vi "data to registers.vi"(6 "word order":T1, 9 "specifications":T2[](array[typedef]), 10 "allocation":u16[](array[numeric]), 11 "data table":T4) -> (2 "registers":u16[](array[numeric]), 3 "allocation":T4)   [LabVIEW 2015, in "Modbus Module runtime.lvclass"]
uses:
  Modbus Module runtime.lvclass
  <vilib>/NI/Tag Bus/table/data table.ctl
  data mapping elements.ctl
  <vilib>/NI/Tag Bus/tag/Data Type.ctl
  <vilib>/NI/Tag Bus/table/data polymorphs/read one/read Double.vi
  <vilib>/NI/Tag Bus/table/data polymorphs/read one/read Single.vi
  <vilib>/NI/Tag Bus/table/data polymorphs/read one/read I64.vi
  <vilib>/NI/Tag Bus/table/data polymorphs/read one/read U64.vi
  <vilib>/NI/Tag Bus/table/data polymorphs/read one/read I32.vi
  <vilib>/NI/Tag Bus/table/data polymorphs/read one/read U32.vi
  <vilib>/NI/Tag Bus/table/data polymorphs/read one/read I16.vi
  <vilib>/NI/Tag Bus/table/data polymorphs/read one/read U16.vi
  <vilib>/NI/Tag Bus/table/data polymorphs/read one/read I8.vi
  <vilib>/NI/Tag Bus/table/data polymorphs/read one/read U8.vi
  <vilib>/NI/Tag Bus/table/data polymorphs/read one/read String.vi
  <vilib>/NI/Tag Bus/table/data polymorphs/read one/read Boolean.vi
  <vilib>/NI/Tag Bus/table/data table.lvlib
  <vilib>/NI/Tag Bus/tag/tag descriptor.lvclass
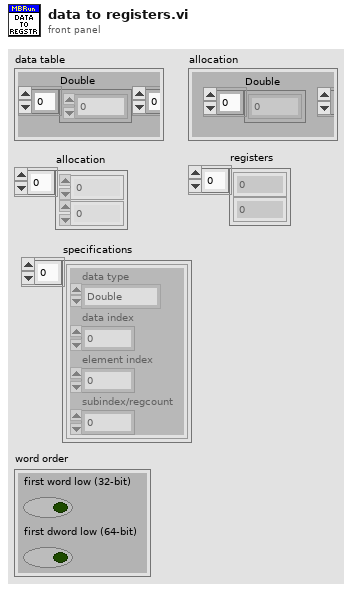
[diagram p1: front panel]
types:
  T1 = cluster{"first word low (32-bit)":bool, "first dword low (64-bit)":bool}
  T2 = typedef "Modbus Module runtime.lvclass/data mapping elements.ctl" = cluster{"data type":T3, "data index":i32, "element index":i32, "subindex/regcount":i32}
  T3 = typedef "tag bus.lvlib/tag descriptor.lvclass/Data Type.ctl" = enum16{"Double", "Single", "I64", "I32", "I16", "I8", "U64", "U32", "U16", "U8", "Boolean", "String", "Array of Double", "Array of Single", "Array of I64", "Array of I32", "Array of I16", "Array of I8", "Array of U64", "Array of U32", "Array of U16", "Array of U8", "Array of Boolean", "Array of String"}
  T4 = typedef "tag bus.lvlib/data table.lvlib/data table.ctl" = cluster{"Double":dbl[], "Single":sgl[], "I64":i64[], "I32":i32[], "I16":i16[], "I8":i8[], "U64":u64[], "U32":u32[], "U16":u16[], "U8":u8[], "Boolean":bool[], "String":string[], "Array of Double":cluster{"DBL Array":dbl[]}[], "Array of Single":cluster{"SGL Array":sgl[]}[], "Array of I64":cluster{"I64 Array":i64[]}[], "Array of I32":cluster{"I32 Array":i32[]}[], "Array of I16":cluster{"I16 Array":i16[]}[], "Array of I8":cluster{"I8 Array":i8[]}[], "Array of U64":cluster{"U64 Array":u64[]}[], "Array of U32":cluster{"U32 Array":u32[]}[], "Array of U16":cluster{"U16 Array":u16[]}[], "Array of U8":cluster{"U8 Array":u8[]}[], "Array of Boolean":cluster{"Boolean Array":bool[]}[], "Array of String":cluster{"String Array":string[]}[]}
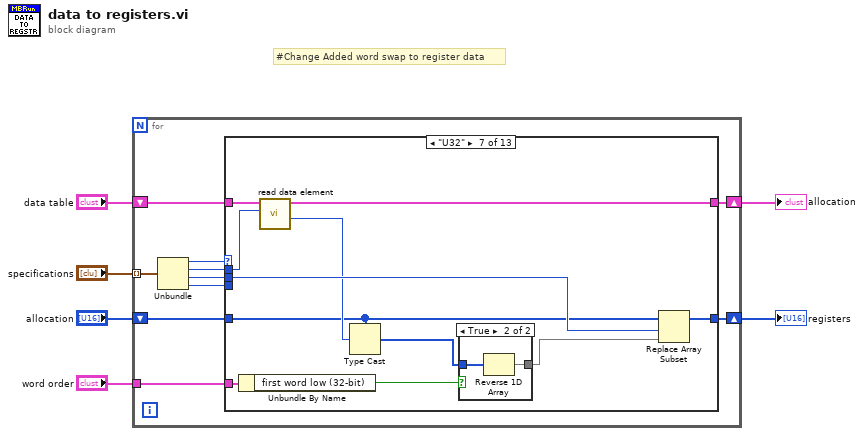
[diagram p0: block diagram]
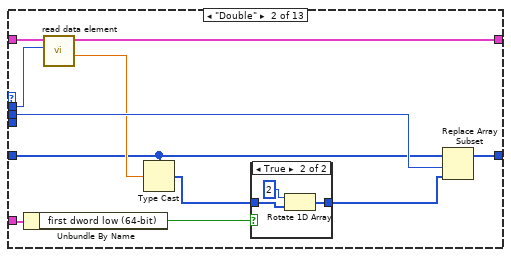
[diagram p3: hidden frame]
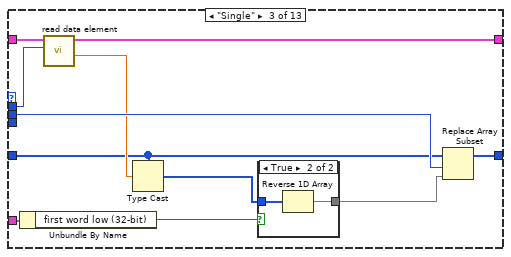
[diagram p5: hidden frame]
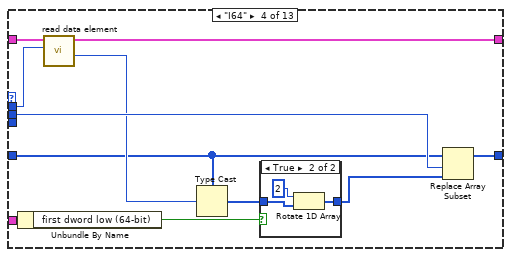
[diagram p7: hidden frame]
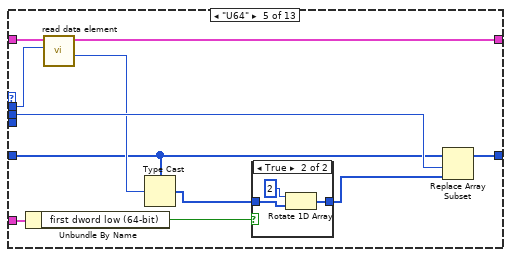
[diagram p9: hidden frame]
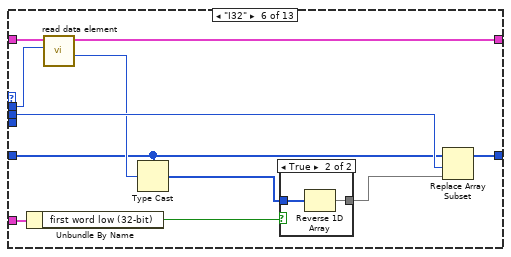
[diagram p11: hidden frame]
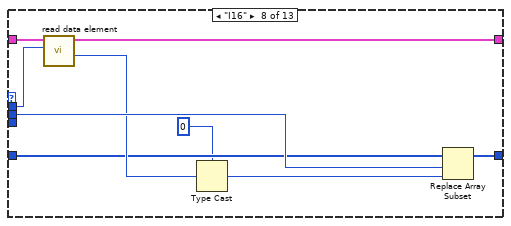
[diagram p14: hidden frame]
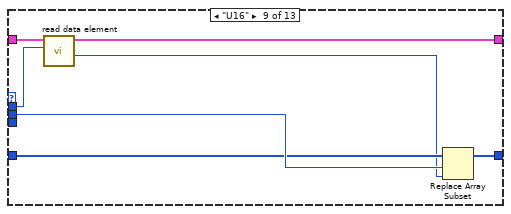
[diagram p15: hidden frame]
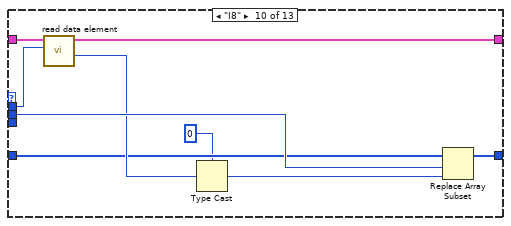
[diagram p16: hidden frame]
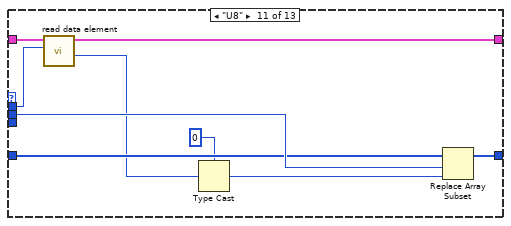
[diagram p17: hidden frame]
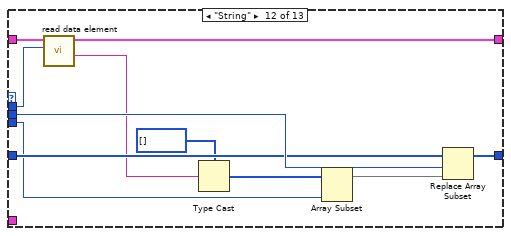
[diagram p18: hidden frame]
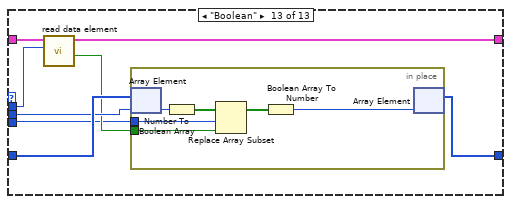
[diagram p19: hidden frame]
diagram:
  # "#Change Added word swap to register data"
  n1 = for {
    shift-right: [w13] -> w5
    shift-left: "data table" -> [w14]
    tunnel: "specifications" -> [w16] mode=indexing
    shift-right: [w9] -> w2
    shift-left: "allocation" -> [w12]
    tunnel: "word order" -> [w7]
    n2 = Unbundle(w16) -> ("data type"=w15:T3, "data index"=w11:i32, "element index"=w8:i32, "subindex/regcount"=w10:i32)
    n3 = case shown="\"U32\"" w15 {
      tunnel: w14 -> [w18 w29 w44 w58 w73 w88 w102 w114 w121 w130 w139 w150 w158]
      tunnel: [w18 w28 w43 w57 w72 w87 w101 w113 w120 w129 w138 w149 w157] -> w13
      tunnel: w8 -> [_ w25 w40 w54 w69 w84 w98 w110 w117 w126 w135 w146 w153]
      tunnel: w12 -> [w17 w23 w38 w52 w67 w82 w96 w108 w116 w124 w134 w145 w155]
      tunnel: w11 -> [_ w27 w42 w56 w71 w86 w100 w112 w119 w128 w137 w148 w156]
      tunnel: w10 -> [_ _ _ _ _ _ _ _ _ _ _ w140 w151]
      tunnel: [w17 w26 w41 w55 w70 w85 w99 w111 w118 w127 w136 w147 w154] -> w9
      tunnel: w7 -> [_ w22 w35 w51 w64 w81 w93 _ _ _ _ _ _]
      frame Default {
      }
      frame "Double" {
        n4 = Unbundle By Name(w22) -> ("first dword low (64-bit)"=w21:bool)
        n5 = call-poly <vilib>:"read data element.vi"("index"=w27, "data table in"=w29) -> ("value"=w24:dbl, "data table out"=w28:T4)  [unwired: 8 in]
        n6 = Type Cast(type=w23, x=w24) -> (*(type *) &x=w20:u16[])
        n7 = case shown="True" w21 {
          tunnel: w20 -> [w30 w33]
          tunnel: [w30 w32] -> w19
          frame False {
          }
          frame True {
            n8 = Rotate 1D Array(1:w33, 2:2 ("n")) -> (0:w32:u16[])
          }
        }
        n9 = Replace Array Subset(array=w23, new element=w19, index=w25) -> (w26:u16[])
      }
      frame "Single" {
        n10 = Unbundle By Name(w35) -> ("first word low (32-bit)"=w34:bool)
        n11 = call-poly <vilib>:"read data element.vi"("index"=w42, "data table in"=w44) -> ("value"=w39:sgl, "data table out"=w43:T4)  [unwired: 8 in]
        n12 = Type Cast(type=w38, x=w39) -> (*(type *) &x=w37:u16[])
        n13 = case shown="True" w34 {
          tunnel: w37 -> [w45 w47]
          tunnel: [w45 w46] -> w36
          frame False {
          }
          frame True {
            n14 = Reverse 1D Array(array=w47) -> (reversed array=w46:u16[])
          }
        }
        n15 = Replace Array Subset(array=w38, new element=w36, index=w40) -> (w41:u16[])
      }
      frame "I64" {
        n16 = Unbundle By Name(w51) -> ("first dword low (64-bit)"=w50:bool)
        n17 = call-poly <vilib>:"read data element.vi"("index"=w56, "data table in"=w58) -> ("value"=w53:i64, "data table out"=w57:T4)  [unwired: 8 in]
        n18 = Type Cast(type=w52, x=w53) -> (*(type *) &x=w49:u16[])
        n19 = case shown="True" w50 {
          tunnel: w49 -> [w59 w62]
          tunnel: [w59 w61] -> w48
          frame False {
          }
          frame True {
            n20 = Rotate 1D Array(1:w62, 2:2 ("n")) -> (0:w61:u16[])
          }
        }
        n21 = Replace Array Subset(array=w52, new element=w48, index=w54) -> (w55:u16[])
      }
      frame "U64" {
        n22 = Unbundle By Name(w64) -> ("first dword low (64-bit)"=w63:bool)
        n23 = call-poly <vilib>:"read data element.vi"("index"=w71, "data table in"=w73) -> ("value"=w68:u64, "data table out"=w72:T4)  [unwired: 8 in]
        n24 = Type Cast(type=w67, x=w68) -> (*(type *) &x=w66:u16[])
        n25 = case shown="True" w63 {
          tunnel: w66 -> [w74 w77]
          tunnel: [w74 w76] -> w65
          frame False {
          }
          frame True {
            n26 = Rotate 1D Array(1:w77, 2:2 ("n")) -> (0:w76:u16[])
          }
        }
        n27 = Replace Array Subset(array=w67, new element=w65, index=w69) -> (w70:u16[])
      }
      frame "I32" {
        n28 = Unbundle By Name(w81) -> ("first word low (32-bit)"=w80:bool)
        n29 = call-poly <vilib>:"read data element.vi"("index"=w86, "data table in"=w88) -> ("value"=w83:i32, "data table out"=w87:T4)  [unwired: 8 in]
        n30 = Type Cast(type=w82, x=w83) -> (*(type *) &x=w79:u16[])
        n31 = case shown="True" w80 {
          tunnel: w79 -> [w89 w91]
          tunnel: [w89 w90] -> w78
          frame False {
          }
          frame True {
            n32 = Reverse 1D Array(array=w91) -> (reversed array=w90:u16[])
          }
        }
        n33 = Replace Array Subset(array=w82, new element=w78, index=w84) -> (w85:u16[])
      }
      frame "U32" {
        n34 = Unbundle By Name(w93) -> ("first word low (32-bit)"=w92:bool)
        n35 = call-poly <vilib>:"read data element.vi"("index"=w100, "data table in"=w102) -> ("value"=w97:u32, "data table out"=w101:T4)  [unwired: 8 in]
        n36 = Type Cast(type=w96, x=w97) -> (*(type *) &x=w95:u16[])
        n37 = case shown="True" w92 {
          tunnel: w95 -> [w103 w105]
          tunnel: [w103 w104] -> w94
          frame False {
          }
          frame True {
            n38 = Reverse 1D Array(array=w105) -> (reversed array=w104:u16[])
          }
        }
        n39 = Replace Array Subset(array=w96, new element=w94, index=w98) -> (w99:u16[])
      }
      frame "I16" {
        n40 = call-poly <vilib>:"read data element.vi"("index"=w112, "data table in"=w114) -> ("value"=w109:i16, "data table out"=w113:T4)  [unwired: 8 in]
        n41 = Type Cast(type=u16 0, x=w109) -> (*(type *) &x=w107:u16)
        n42 = Replace Array Subset(array=w108, new element=w107, index=w110) -> (w111:u16[])
      }
      frame "U16" {
        n43 = call-poly <vilib>:"read data element.vi"("index"=w119, "data table in"=w121) -> ("value"=w115:u16, "data table out"=w120:T4)  [unwired: 8 in]
        n44 = Replace Array Subset(array=w116, new element=w115, index=w117) -> (w118:u16[])
      }
      frame "I8" {
        n45 = call-poly <vilib>:"read data element.vi"("index"=w128, "data table in"=w130) -> ("value"=w125:i8, "data table out"=w129:T4)  [unwired: 8 in]
        n46 = Type Cast(type=u16 0, x=w125) -> (*(type *) &x=w123:u16)
        n47 = Replace Array Subset(array=w124, new element=w123, index=w126) -> (w127:u16[])
      }
      frame "U8" {
        n48 = call-poly <vilib>:"read data element.vi"("index"=w137, "data table in"=w139) -> ("value"=w133:u8, "data table out"=w138:T4)  [unwired: 8 in]
        n49 = Type Cast(type=u16 0, x=w133) -> (*(type *) &x=w132:u16)
        n50 = Replace Array Subset(array=w134, new element=w132, index=w135) -> (w136:u16[])
      }
      frame "String" {
        n51 = call-poly <vilib>:"read data element.vi"("index"=w148, "data table in"=w150) -> ("value"=w144:string, "data table out"=w149:T4)  [unwired: 8 in]
        n52 = Type Cast(type=u16[] [] ("allocation"), x=w144) -> (*(type *) &x=w143:u16[])
        n53 = Array Subset(array=w143, length=w140) -> (w141:u16[])  [unwired: 1 in]
        n54 = Replace Array Subset(array=w145, new element=w141, index=w146) -> (w147:u16[])
      }
      frame "Boolean" {
        n55 = call-poly <vilib>:"read data element.vi"("index"=w156, "data table in"=w158) -> ("value"=w152:bool, "data table out"=w157:T4)  [unwired: 8 in]
        n56 = in-place {
          in-place-border: w152 -> [w160]
          in-place-border: w151 -> [w159]
          n57 = in-place-array #1(w155, w153) -> (w164:u16)
          n58 = Number To Boolean Array(number=w164) -> (Boolean array=w162:bool[])
          n59 = Replace Array Subset(array=w162, new element=w160, index=w159) -> (w161:bool[])
          n60 = Boolean Array To Number(Boolean array=w161) -> (number=w163:u16)
          n61 = in-place-array #1(w163) -> (w154:u16[])  [unwired: 1 out]
        }
      }
    }
  }
  "allocation" <- w5
  "registers" <- w2
